vi "SF_Servo.vi"() -> ()   [LabVIEW 2021]
uses:
  <vilib>/Simulation/Scripting/Companion Diagram/SimConfigNode/SimParams.ctl
  <vilib>/Simulation/Scripting/Companion Diagram/SimConfigNode/_simSolvers.ctl
  <vilib>/Simulation/Implementation/Shared/SIMSCR Execution Mode.ctl
  <vilib>/Simulation/Param Hierarchy/Typedefs/SIMPH Param Control Actions.ctl
  <vilib>/Simulation/Implementation/Shared/NILVSim_ParamChanged.vi
  <vilib>/Simulation/Implementation/Shared/NILVSIM_BeginStep.vi
  <vilib>/Simulation/DataSources/Implementation/NILVSim Step.llb/SIM Step (scalar).vi
  <vilib>/Simulation/ContinuousLinear/Implementation/NILVSim State Space.llb/SIM State Space Distributor (CD).vi
  <vilib>/Simulation/SignalDisplay/Implementation/NILVSim Time Waveform.llb/SIM Time Waveform (scalar).vi
  <vilib>/Simulation/SignalArithmetic/Implementation/NILVSim Gain.llb/SIM Gain (vector,MatrixGain).vi
  <vilib>/Simulation/SignalDisplay/Implementation/NILVSim Time Waveform.llb/SIM Time Waveform (vector).vi
  <vilib>/Simulation/SignalArithmetic/Implementation/NILVSim Gain.llb/SIM Gain (scalar).vi
  <vilib>/Simulation/ContinuousLinear/Implementation/NILVSim State Space.llb/SIM State Space Collector (CD).vi
  <vilib>/Simulation/Implementation/Shared/NILVSim_Manager.vi
  <vilib>/Utility/error.llb/Clear Errors.vi
  <vilib>/Simulation/Implementation/Shared/NILVSim_FinalizeModel.vi
  <vilib>/addons/Control Design/_Model Construction/Model Creation.llb/Model Creation SubVI/cd_Create State Space Model.vi
  <vilib>/addons/Control Design/_Dynamic Analysis/Dynamic Analysis.llb/Dynamic Analysis subVI/cd_Poles (State-Space).vi
  <vilib>/addons/Control Design/_Utility/Model Viewer.llb/Model Viewer SubVI/cd_Draw State-Space Equation (SS).vi
  <vilib>/Simulation/Implementation/Shared/SIM Unbundle Sim Info.vi
  <vilib>/Simulation/Implementation/Shared/NILVSim_Initialize.vi
  <vilib>/Simulation/Utility/Implementation/NILVSim Get Time and IsAcceptedStep.vi
  <vilib>/Simulation/Implementation/Shared/SIMSH Read Queue.vi
  <vilib>/Simulation/Implementation/Shared/NILVSim_GetModelError.vi
  <vilib>/Simulation/Implementation/Shared/SIM Bundle Sim Info.vi
  <vilib>/Simulation/Scripting/Companion Diagram/SimConfigNode/SimDog.xnode
  <vilib>/Simulation/Implementation/XNodeFramework/SimXNode/SimX.xnode
  <vilib>/addons/Control Design/_Model Construction/NI_LinSys_Model Creation.lvlib
  <vilib>/addons/Control Design/_Utility/NI_CD_Model Viewer.lvlib
  <vilib>/addons/Control Design/_Dynamic Analysis/NI_CD_Dynamic Analysis.lvlib
  <vilib>/addons/Control Design/_State-Space Analysis/NI_CD_State-Space Analysis.lvlib
  <vilib>/addons/Control Design/_Model Construction/Model Typedefs.llb/CD General Elements.ctl
  <vilib>/addons/Control Design/_Model Construction/NI_LinSys_Model Typedefs.lvlib
  <vilib>/addons/Control Design/_Model Construction/Model Typedefs.llb/CD State Space Model (MIMO).ctl
  <vilib>/Simulation/ContinuousLinear/Implementation/NILVSim State Space.llb/SIM State Space (CD).vi
  <vilib>/Simulation/Implementation/Shared/NI_SIM_Implementation.lvlib
panel:
  out "State-Feedback Gain":dbl[][](array[numeric])=[[0.6994266666666668, 0.2800000000000001]] format="%.2f"
  in  "?":dbl[][](array[numeric])=[[0.0, -3405.44, -674.22, -717.74]] format="%#.5g"
  in  "K1":dbl=-2657.24
  in  "Final Time (s)":dbl=1.0
  in  "r":dbl(slide)=0.10204081632653061 scale=-1.0..1.0
  out "Response (theta)":waveform(dbl)[](graph)=[{"t0"=timestamp(1 s since 1904-01-01), "dt"=1.0, "Y"=[0.10204081632653061]}, {"t0"=timestamp(1 s since 1904-01-01), "dt"=1.0, "Y"=[0.10231817434302816]}]
  out "Error":waveform(dbl)(graph)={"t0"=timestamp(1 s since 1904-01-01), "dt"=1.0, "Y"=[-0.00027735801649754477]}
  out "omega":waveform(dbl)(graph)={"t0"=timestamp(1 s since 1904-01-01), "dt"=1.0, "Y"=[-0.000460291339728839]}
  out "Is Controllable?":bool=TRUE
  out "Controllability Matrix":dbl[][](array[numeric])=[[0.0, 1.0, 0.0, 2.45], [0.0, -1.0, 0.0, -12.26], [1.0, 0.0, 2.45, 0.0], [-1.0, 0.0, -12.26, 0.0]] format="%.2f"
  out "Open Loop Poles":cdb[](array[numeric])=[3.5014282800023193+0.0i, -3.5014282800023193+0.0i, 0.0+0.0i, 0.0+0.0i] format="%.3f"
  out "Equation":picture
  in  "D":dbl[][](array[numeric])=[[0.0]] format="%#.5g"
  in  "C":dbl[][](array[numeric])=[[1.0, 0.0, 0.0, 0.0]] format="%#.5g"
  in  "B":dbl[][](array[numeric])=[[0.0], [0.0], [1.0], [-1.0]] format="%#.5g"
  in  "A":dbl[][](array[numeric])=[[0.0, 0.0, 1.0, 0.0], [0.0, 0.0, 0.0, 1.0], [0.0, -2.45, 0.0, 0.0], [0.0, 12.26, 0.0, 0.0]] format="%#.5g"
  out "A(4,2)":dbl=12.262500000000001
  out "B(4,1)":dbl=-1.0
  in  "L":dbl=1.0
  out "B(3,1)":dbl=1.0
  in  "M":dbl=1.0
  in  "g":dbl=9.81
  in  "m":dbl=0.25
  out "A(3,2)":dbl=-2.4525
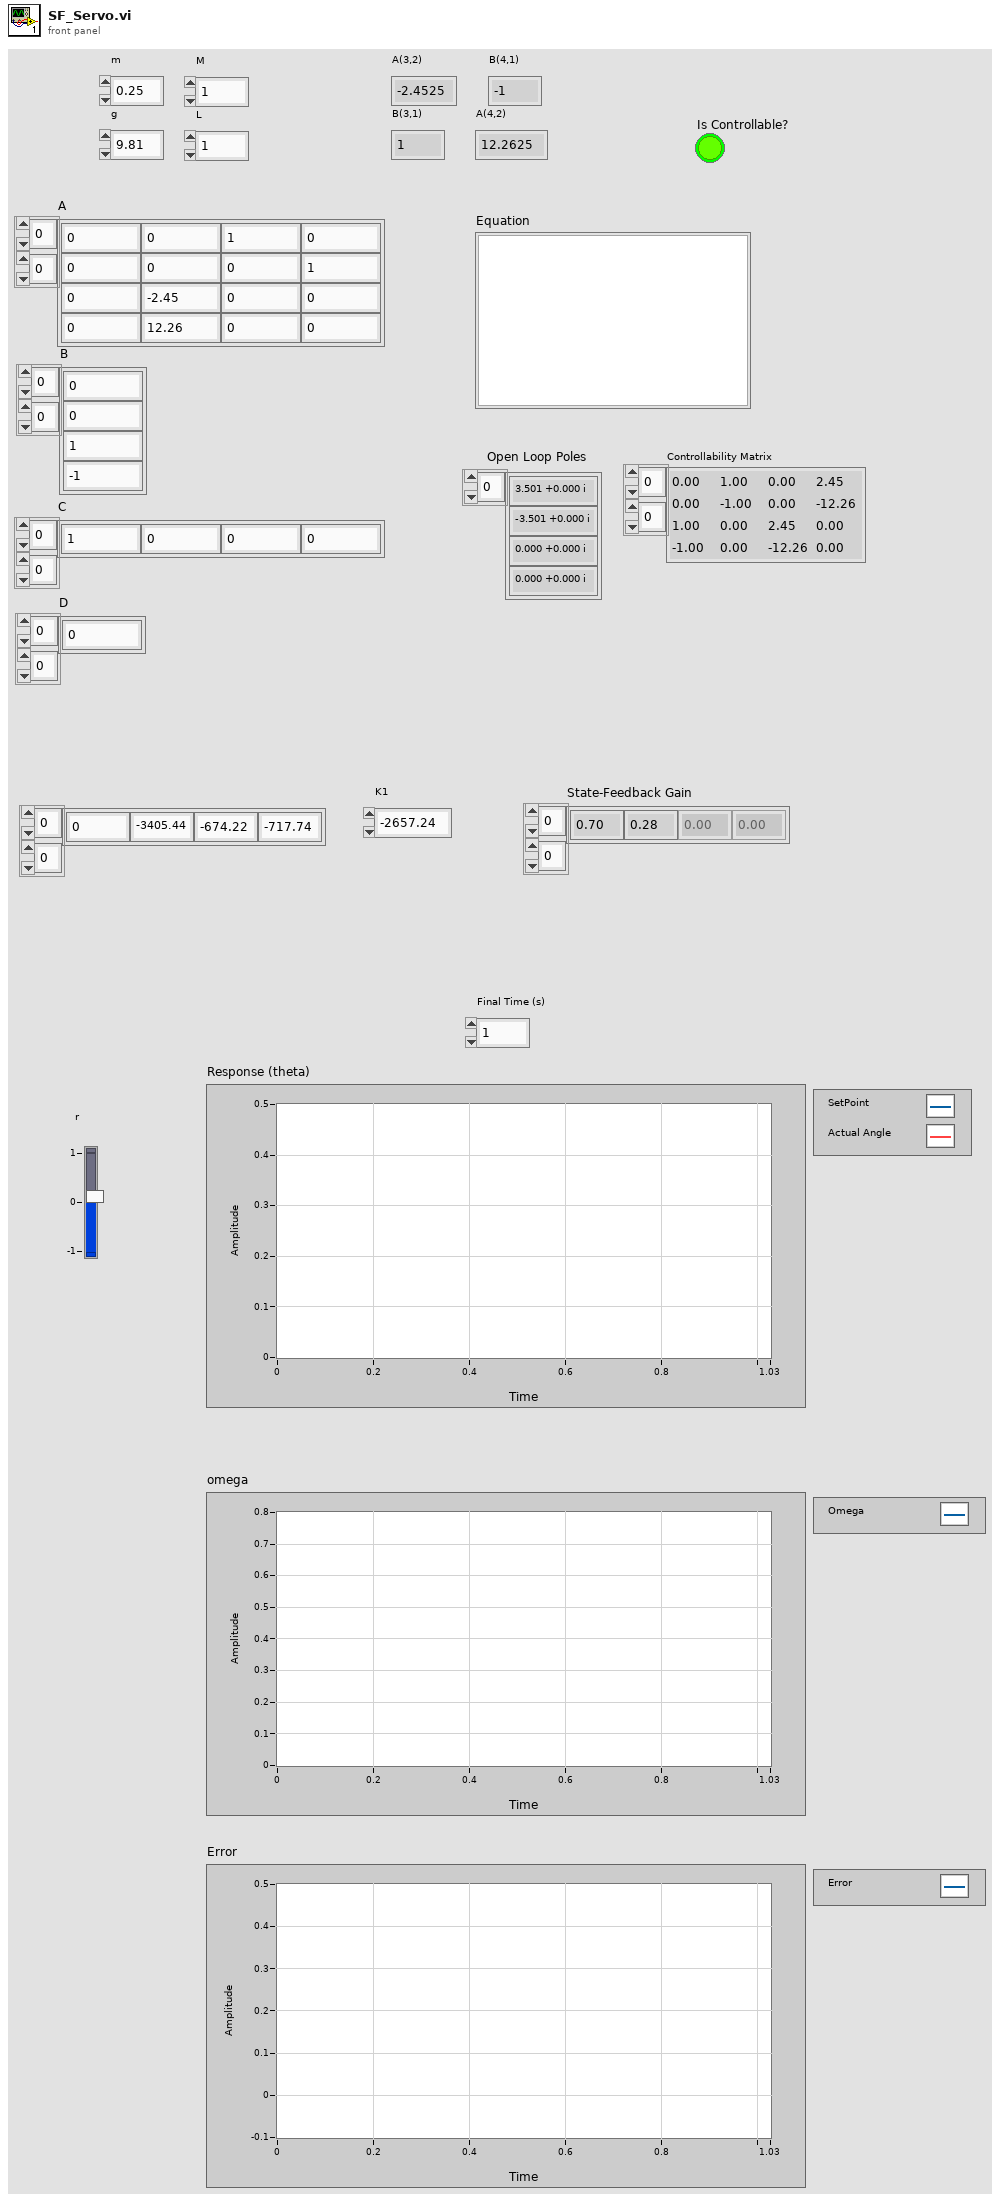
[diagram p1: front panel]
types:
  T1 = typedef "NI_LinSys_Model Typedefs.lvlib/CD State Space Model (MIMO).ctl" = cluster{"properties":T2, "A":dbl[][], "B":dbl[][], "C":dbl[][], "D":dbl[][], "StateNames":string[], "Transport Delay":dbl[][]}
  T2 = typedef "NI_LinSys_Model Typedefs.lvlib/CD General Elements.ctl" = cluster{"Model name":string, "Input names":string[], "Output names":string[], "Input Delays":dbl[], "Output Delays":dbl[], "Sampling Time":dbl, "Notes":string}
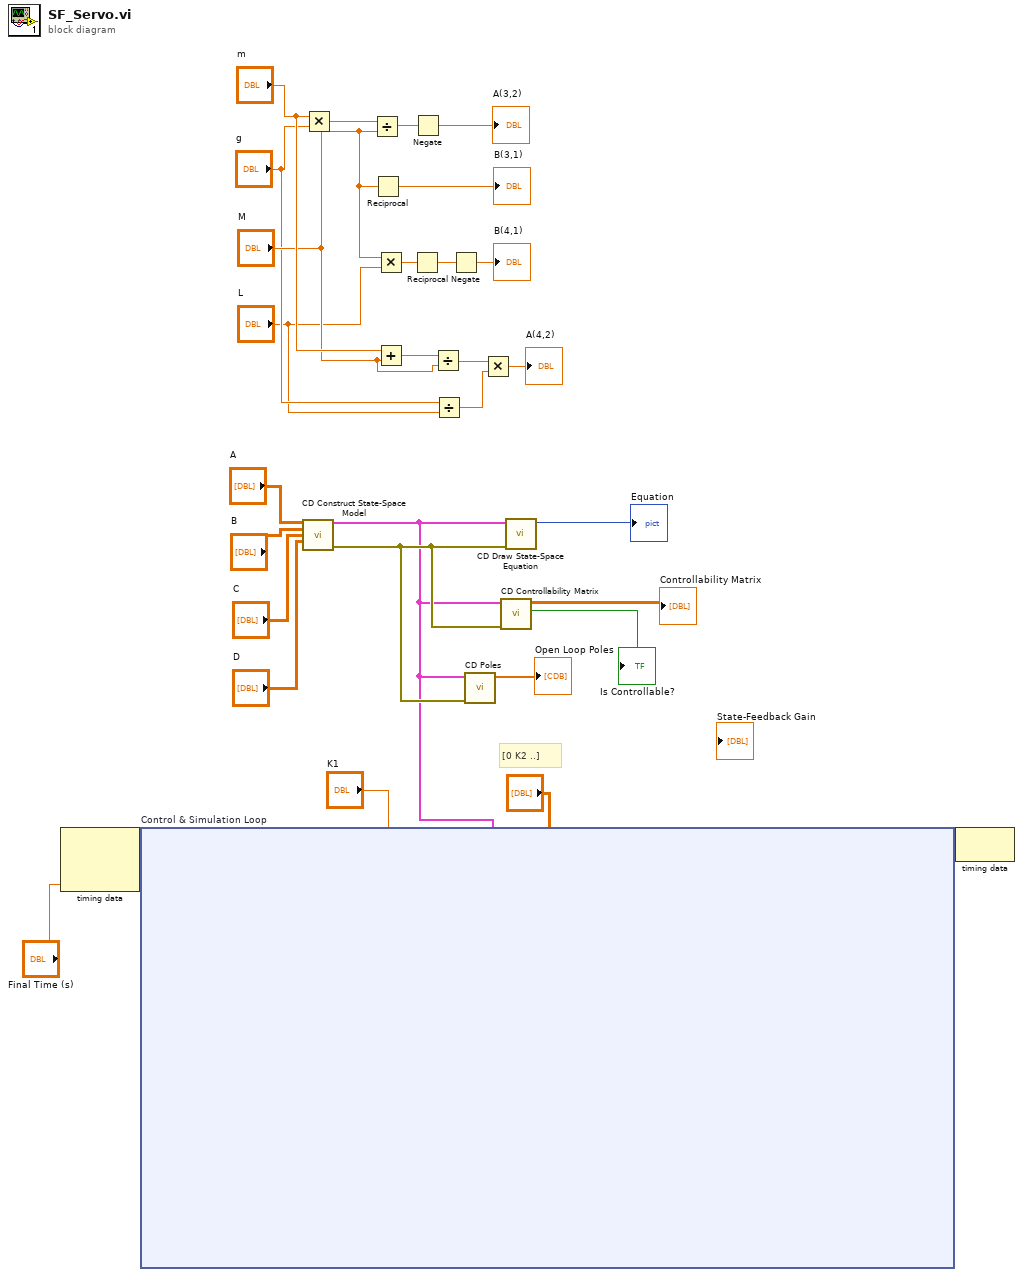
[diagram p0: block diagram]
diagram:
  # "[0 K2 ..]"
  n1 = node-c288("Final Time (s)") -> (w30:variant)  [unwired: 2 in]
  n2 = call-poly <vilib>:"CD Construct State-Space Model.vi"("A"="A", "B"="B", "C"="C", "D"="D") -> ("State-Space Model"=w2:T1, "error out"=w8:errorcluster)  [unwired: 10 in]
  n3 = node-c254 "Control & Simulation Loop"(w30, "K1", w2, "?") -> (w29:variant)
  n4 = Multiply(x="m", y="g") -> (x*y=w27:dbl)
  n5 = Divide(x=w27, y="M") -> (x/y=w28:dbl)
  n6 = Reciprocal(x="M") -> (1/x=→"B(3,1)":dbl)
  n7 = Multiply(x="M", y="L") -> (x*y=w23:dbl)
  n8 = Add(x="m", y="M") -> (x+y=w20:dbl)
  n9 = Reciprocal(x=w23) -> (1/x=w24:dbl)
  n10 = Negate(x=w28) -> (-x=→"A(3,2)":dbl)
  n11 = Divide(x=w20, y="M") -> (x/y=w18:dbl)
  n12 = Divide(x="g", y="L") -> (x/y=w15:dbl)
  n13 = Negate(x=w24) -> (-x=→"B(4,1)":dbl)
  n14 = call-poly <vilib>:"CD Poles.vi"("error in (no error)"=w8, "State-Space Model"=w2) -> ("Poles"=→"Open Loop Poles":cdb[])  [unwired: 8 in, 1 out]
  n15 = Multiply(x=w18, y=w15) -> (x*y=→"A(4,2)":dbl)
  n16 = call <vilib>:"CD Controllability Matrix.vi"("error in (no error)"=w8, "State-Space Model"=w2) -> ("Is Controllable?"=→"Is Controllable?":bool, "Controllability Matrix"=→"Controllability Matrix":dbl[][])  [unwired: 6 in, 2 out]
  n17 = call-poly <vilib>:"CD Draw State-Space Equation.vi"("error in (no error)"=w8, "State-Space Model"=w2) -> ("Equation"=→"Equation":picture)  [unwired: 7 in, 2 out]
  n18 = node-c288(w29) -> ()  [unwired: 1 out]
